vi "KG set pump control.vi"(8 "Fehler (Eingang, kein Fehler)":errorcluster, 10 "control mode":u32, 11 "VISA-Ressourcenname":refnum<visa-resource-name>) -> (0 "Fehler (Ausgang)":errorcluster, 2 "Komando gesedet":string, 3 "VISA-Ressourcenname (Ausgang)":refnum<visa-resource-name>)   [LabVIEW 2020, in "Linearisierung v2.lvlib" / "Gasteiler.lvlib" / "HovaCAL_Interface.lvlib" / "KGN.lvlib" / "set.lvlib"]
uses:
  set.lvlib
  KGN.lvlib
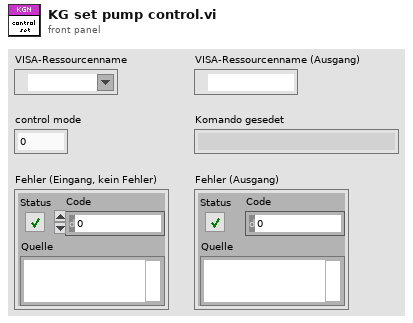
[diagram p1: front panel]
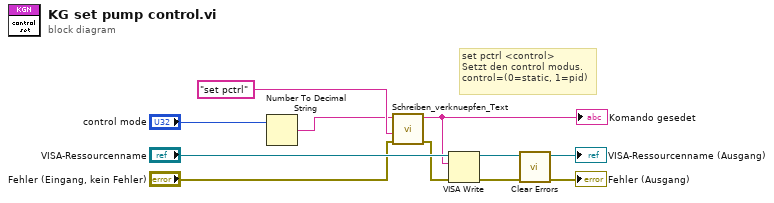
[diagram p0: block diagram]
diagram:
  # "set pctrl <control>\nSetzt den control modus.\ncontrol=(0=static, 1=pid)"
  n1 = Number To Decimal String(number="control mode") -> (decimal integer string=w3:string)  [unwired: 1 in]
  n2 = call "Schreiben_verknuepfen_Text.vi"("error in (no error)"="Fehler (Eingang, kein Fehler)", "Order"="set pctrl" ("Schreibpuffer"), "parameter"=w3) -> ("error out"=w6:errorcluster, "Verknüpfter String"=w5:string)  [unwired: 7 in]
  "Komando gesedet" <- w5
  n3 = VISA Write(VISA resource name="VISA-Ressourcenname", write buffer=w5, error in (no error)=w6) -> (VISA resource name out=→"VISA-Ressourcenname (Ausgang)":refnum<visa-resource-name>, error out=w2:errorcluster)  [unwired: 1 out]
  n4 = call <vilib>:"Clear Errors.vi"("error in (no error)"=w2) -> ("error out"=→"Fehler (Ausgang)":errorcluster)  [unwired: 5 in, 1 out]
